vi "PathPlanner_Trajectory_GetWPITrajectory.vi"(11 "PathPlannerTrajectory":T7 {"States"."TargetHolonomicRotation"."SIN" format="%13.4f"; "States"."TargetHolonomicRotation"."COS" format="%13.4f"; "States"."TargetHolonomicRotation"."VALUE" format="%13.4f"; "States"."Heading"."SIN" format="%13.4f"; "States"."Heading"."COS" format="%13.4f"; "States"."Heading"."VALUE" format="%13.4f"; "States"."PositionMeters"."Y" format="%14.3f"; "States"."PositionMeters"."X" format="%14.3f"}) -> (1 "WPITrajHolonomicPoses":T1[](array[typedef]) {"HolonomicPose"."ROTATION"."SIN" format="%13.4f"; "HolonomicPose"."ROTATION"."COS" format="%13.4f"; "HolonomicPose"."ROTATION"."VALUE" format="%13.4f"; "HolonomicPose"."TRANSLATION"."Y" format="%14.3f"; "HolonomicPose"."TRANSLATION"."X" format="%14.3f"}, 3 "TRAJECTORY":T5 {"States"."POSE"."ROTATION"."SIN" format="%13.4f"; "States"."POSE"."ROTATION"."COS" format="%13.4f"; "States"."POSE"."ROTATION"."VALUE" format="%13.4f"; "States"."POSE"."TRANSLATION"."Y" format="%14.3f"; "States"."POSE"."TRANSLATION"."X" format="%14.3f"; "TotalTImeSecs" format="%20.3f"})   [LabVIEW 2019, in "PathPlanner24.lvlib"]
doc: "Convert a PathPlanner trajectory into a LabVIEW / WPILib Trajectory. \n\nInputs:\n -- PathPlannerTrajectory -- PathPlanner Trajectory data cluster\n\nOutputs\n -- Traectory -- LabVIEW traectory library (WPlib style) trajectory data cluster."
uses:
  PathPlanner24.lvlib
  TypeDef/PathPlannerTrajectory.ctl
  TypeDef/PathPlannerTrajectoryState.ctl
  <vilib>/Rock Robotics/WPI/ThirdParty/JAS_Junk/TrajLib/TypeDef/TRANSLATION2D.ctl
  <vilib>/Rock Robotics/WPI/ThirdParty/JAS_Junk/TrajLib/TypeDef/ROTATION2D.ctl
  TypeDef/PathPlannerPathConstraints.ctl
  <vilib>/Rock Robotics/WPI/ThirdParty/JAS_Junk/TrajLib/TypeDef/TRAJECTORY.ctl
  <vilib>/Rock Robotics/WPI/ThirdParty/JAS_Junk/TrajLib/TypeDef/TRAJ_STATE.ctl
  <vilib>/Rock Robotics/WPI/ThirdParty/JAS_Junk/TrajLib/TypeDef/POSE2D.ctl
  TypeDef/PathPlannerWPITrajHolonomicPose.ctl
  <vilib>/Rock Robotics/WPI/ThirdParty/JAS_Junk/TrajLib/TrajectoryState_New.vi
  <vilib>/Rock Robotics/WPI/ThirdParty/JAS_Junk/TrajLib/Pose2d_New_TRRO.vi
  <vilib>/Rock Robotics/WPI/ThirdParty/JAS_Junk/TrajLib/Trajectory_Library.lvlib
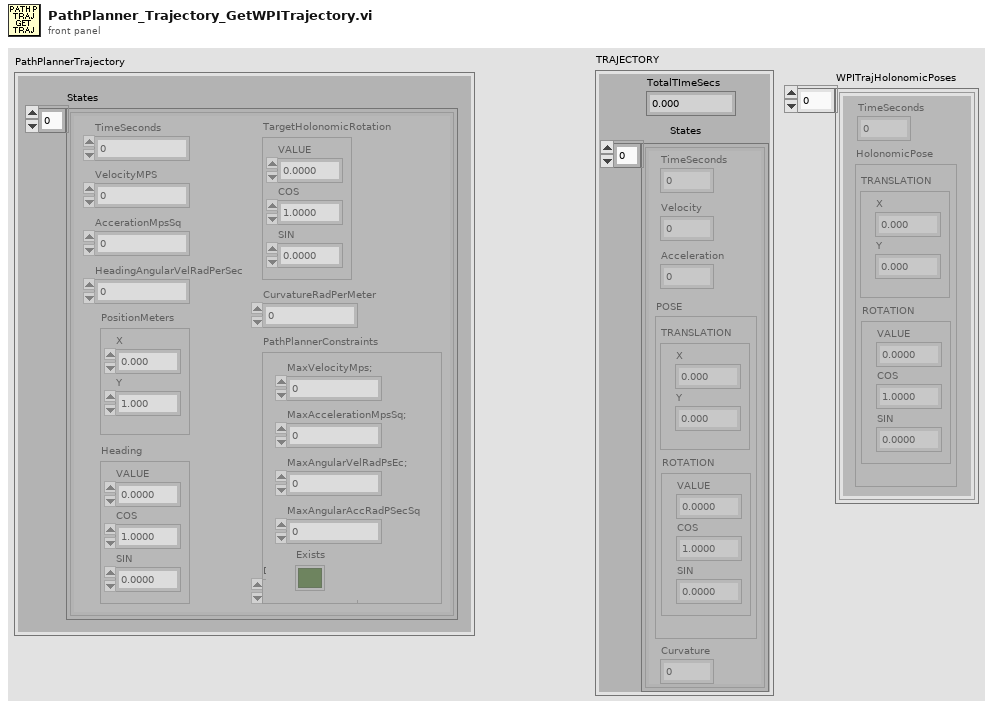
[diagram p1: front panel]
types:
  T1 = typedef "PathPlanner24.lvlib/PathPlannerWPITrajHolonomicPose.ctl" = cluster{"TimeSeconds":dbl, "HolonomicPose":T2}
  T2 = typedef "Trajectory_Library.lvlib/POSE2D.ctl" = cluster{"TRANSLATION":T3, "ROTATION":T4}
  T3 = typedef "Trajectory_Library.lvlib/TRANSLATION2D.ctl" = cluster{"X":dbl, "Y":dbl}
  T4 = typedef "Trajectory_Library.lvlib/ROTATION2D.ctl" = cluster{"VALUE":dbl, "COS":dbl, "SIN":dbl}
  T5 = typedef "Trajectory_Library.lvlib/TRAJECTORY.ctl" = cluster{"TotalTImeSecs":dbl, "States":T6[]}
  T6 = typedef "Trajectory_Library.lvlib/TRAJ_STATE.ctl" = cluster{"TimeSeconds":dbl, "Velocity":dbl, "Acceleration":dbl, "POSE":T2, "Curvature":dbl}
  T7 = typedef "PathPlanner24.lvlib/PathPlannerTrajectory.ctl" = cluster{"States":T8[]}
  T8 = typedef "PathPlanner24.lvlib/PathPlannerTrajectoryState.ctl" = cluster{"TimeSeconds":dbl, "VelocityMPS":dbl, "AccerationMpsSq":dbl, "HeadingAngularVelRadPerSec":dbl, "PositionMeters":T3, "Heading":T4, "TargetHolonomicRotation":T4, "CurvatureRadPerMeter":dbl, "DeltaPos":dbl, "PathPlannerConstraints":T9}
  T9 = typedef "PathPlanner24.lvlib/PathPlannerPathConstraints.ctl" = cluster{"MaxVelocityMps;":dbl, "MaxAccelerationMpsSq;":dbl, "MaxAngularVelRadPsEc;":dbl, "MaxAngularAccRadPSecSq":dbl, "Exists":bool}
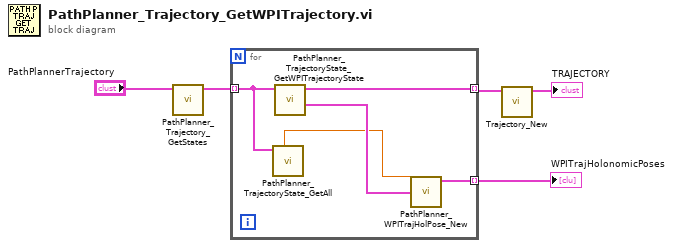
[diagram p0: block diagram]
diagram:
  n1 = call "PathPlanner_Trajectory_GetStates.vi"("PathPlannerTrajectory"="PathPlannerTrajectory") -> ("PathPlannerStates"=w4:T8[])  [unwired: 10 in]
  n2 = for {
    tunnel: w4 -> [w9] mode=indexing
    tunnel: [w10] -> w3 mode=indexing
    tunnel: [w8] -> w1 mode=indexing
    n3 = call "PathPlanner_TrajectoryState_GetAll.vi"("PathPlannerState"=w9) -> ("TimeSeconds"=w6:dbl)  [unwired: 1 in, 9 out]
    n4 = call "PathPlanner_TrajectoryState_GetWPITrajectoryState.vi"("PathPlannerState"=w9) -> ("HolonomicPose"=w7:T2, "TrajectoryState"=w10:T6)  [unwired: 9 in]
    n5 = call "PathPlanner_WPITrajHolPose_New.vi"("HolonomicPose"=w7, "TimeSeconds"=w6) -> ("WPITrajHolonomicPose"=w8:T1)  [unwired: 9 in]
  }
  "WPITrajHolonomicPoses" <- w1
  n6 = call <vilib>:"Trajectory_New.vi"("TRAJ_STATES"=w3) -> ("TRAJECTORY"=→"TRAJECTORY":T5)  [unwired: 10 in]
